vi "monoOpen.vi"(8 "error in":errorcluster) -> (0 "error out":errorcluster, 3 "Mono0ID":u32)   [LabVIEW 2017]
doc: "Retrieves USB handles for the two monochromators"
uses:
  National Instruments/LabVIEW 8.5/vi.lib/cs_USB/cs_USB.lvlib
  Photoinduced Absorption VIs/globalVars.vi
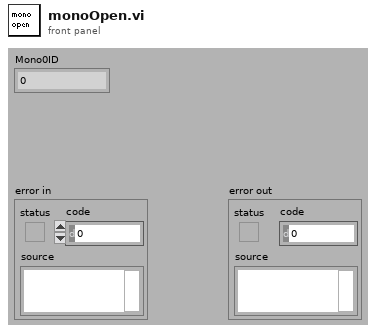
[diagram p1: front panel]
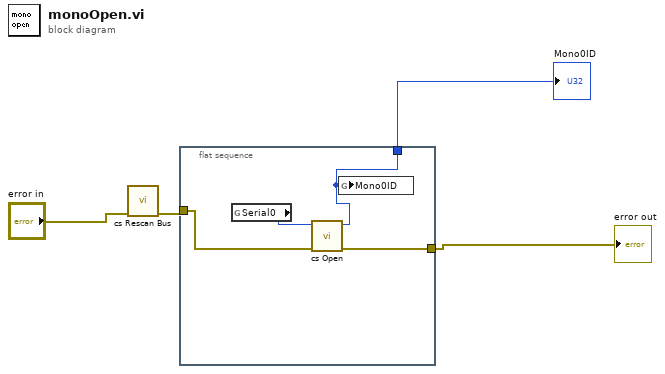
[diagram p0: block diagram]
diagram:
  n1 = call "cs Rescan Bus.vi"("error in (no error)"="error in") -> ("error out"=w2:errorcluster)  [unwired: 10 in]
  n2 = flat-sequence {
    tunnel: w2 -> [w8]
    tunnel: [w6] -> w4
    tunnel: [w5] -> w1
    frame #0 {
      n3 = global read "globalVars.vi" "Serial0"() -> (w7:u32)
      n4 = call "cs Open.vi"("error in (no error)"=w8, "serialNo"=w7) -> ("error out"=w5:errorcluster, "function return"=w6:i32)  [unwired: 8 in]
      n5 = global write "globalVars.vi" "Mono0ID"(w6) -> ()
    }
  }
  "Mono0ID" <- w4
  "error out" <- w1
